vi "Reentrant Send Error.vi"(7 "Queue Names":string[](array[string]), 8 "error in (no error)":errorcluster, 10 "Last State":string, 11 "Queues":refnum<queue>[](array[refnum])) -> (0 "error out":errorcluster)   [LabVIEW 2017]
uses:
  Queue Element.ctl
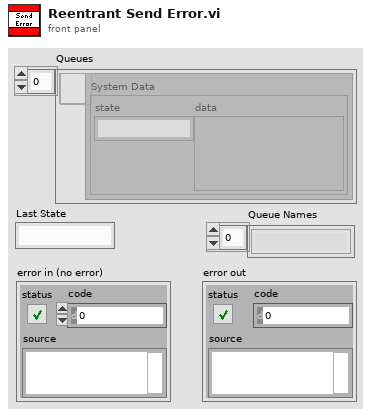
[diagram p1: front panel]
types:
  T1 = typedef "Queue Element.ctl" = cluster{"state":string, "data":variant}
  T2 = cluster{"Last State":string, "error in (no error)":errorcluster}
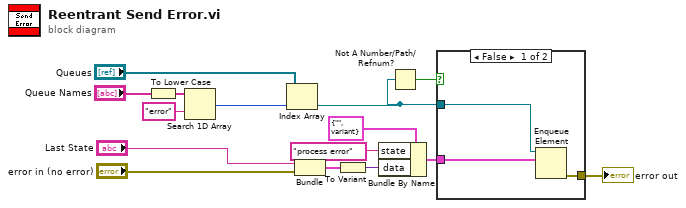
[diagram p0: block diagram]
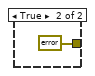
[diagram p2: hidden frame]
diagram:
  n1 = To Lower Case(string="Queue Names") -> (all lower case string=w6:string[])
  n2 = Search 1D Array(1D array=w6, element="error") -> (index of element=w3:i32)  [unwired: 1 in]
  n3 = Index Array(array="Queues", index=w3) -> (element=w2:refnum<queue>)
  n4 = Bundle("Last State"="Last State", "error in (no error)"="error in (no error)") -> (w11:T2)  [unwired: 1 in]
  n5 = To Variant(anything=w11) -> (Variant=w12:variant)
  n6 = Bundle By Name(cluster=T1 {"state"="", "data"=variant} ("System Data"), "state"="process error", "data"=w12) -> (w8:T1)
  n7 = Not A Number/Path/Refnum?(number/path/refnum=w2) -> (NaN/Path/Refnum?=w7:bool)
  n8 = case shown="False" w7 {
    tunnel: [w18 errorcluster {"status"=FALSE, "code"=0, "source"=""} ("error out")] -> w14
    tunnel: w8 -> [w17 _]
    tunnel: w2 -> [w16 _]
    frame False {
      n9 = Enqueue Element(queue=w16, element=w17) -> (error out=w18:errorcluster)  [unwired: 2 in, 2 out]
    }
    frame True {
    }
  }
  "error out" <- w14
